vi "PipelineDuty.vi"(8 "error in (no error)":errorcluster, 10 "DataExchange":T1, 11 "GRMActor in":refnum<class "GenericActor.lvclass">) -> (0 "error out":errorcluster, 2 "DataExchange 2":T1, 3 "GRMActor out":refnum<class "GenericActor.lvclass">)   [LabVIEW 2020, in "GenericActor.lvlib" / "GenericActor.lvclass"]
uses:
  GenericActor.lvclass
  Device/Device/DataExchange.ctl
  Interface/DataListener/DataListener.lvclass
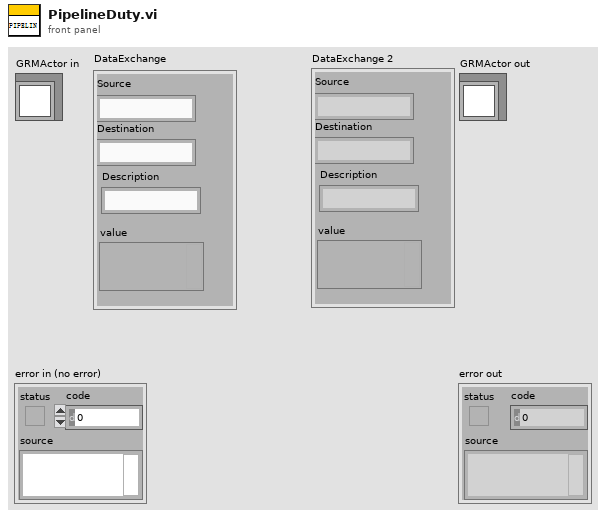
[diagram p1: front panel]
types:
  T1 = typedef "DataListener.lvclass/DataExchange.ctl" = cluster{"Source":string, "Destination":string, "Description":string, "value":variant}
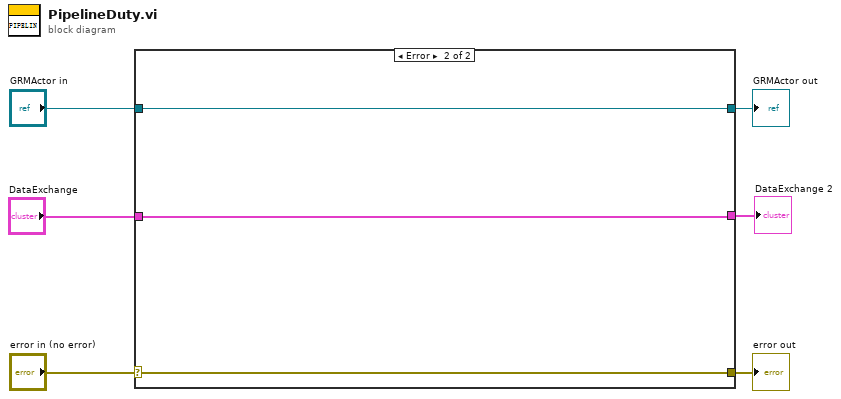
[diagram p0: block diagram]
diagram:
  n1 = case shown="Error" "error in (no error)" {
    selector: "error in (no error)" -> [w8 w12]
    tunnel: [w8 w12] -> w5
    tunnel: [w9 w11] -> w3
    tunnel: "GRMActor in" -> [w9 w11]
    tunnel: [w7 w10] -> w1
    tunnel: "DataExchange" -> [w7 w10]
    frame No Error {
      # "Wire the error cluster across even in the \"No Error\"\ncase so that warnings get propagated."
    }
    frame Error {
    }
  }
  "error out" <- w5
  "GRMActor out" <- w3
  "DataExchange 2" <- w1
